vi "Sort Test Cases.vi"(10 "Test Cases":T1[](array[typedef]), 11 "Test Suites":string[](array[string])) -> (3 "Test Suites":T2[](array[typedef]))   [LabVIEW 2014, in "VI Tester Parsing.lvlib"]
uses:
  VI Tester Parsing.lvlib
  Test Suite.ctl
  Test Case.ctl
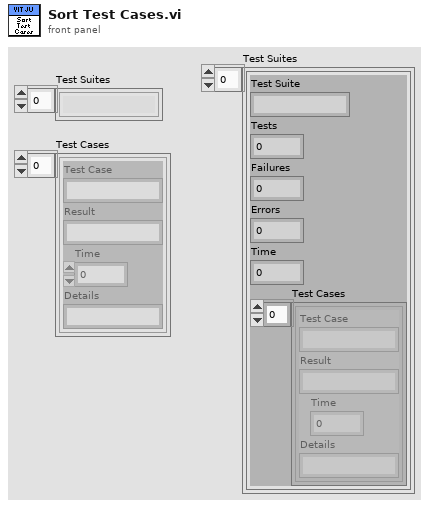
[diagram p1: front panel]
types:
  T1 = typedef "VI Tester Parsing.lvlib/Test Case.ctl" = cluster{"Test Case":string, "Result":string, "Time":dbl, "Details":string}
  T2 = typedef "VI Tester Parsing.lvlib/Test Suite.ctl" = cluster{"Test Suite":string, "Tests":i32, "Failures":i32, "Errors":i32, "Time":dbl, "Test Cases":T1[]}
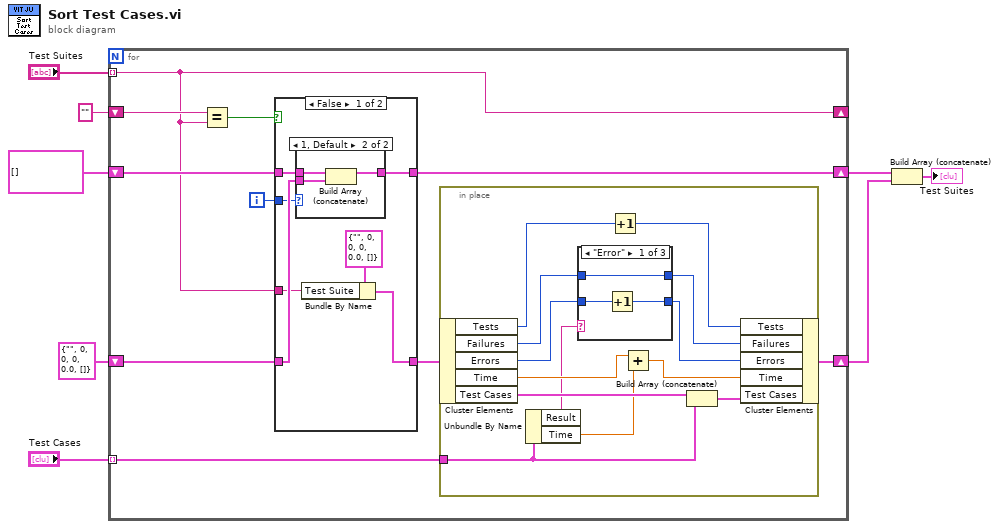
[diagram p0: block diagram]
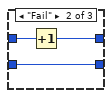
[diagram p2: hidden frame]
diagram:
  n1 = for {
    tunnel: "Test Cases" -> [w17] mode=indexing
    shift-right: [w9] -> _
    shift-left: "" -> [w10]
    shift-right: [w11] -> w6
    shift-left: T2 {"Test Suite"="", "Tests"=0, "Failures"=0, "Errors"=0, "Time"=0.0, "Test Cases"=[]} ("cluster") -> [w16]
    tunnel: "Test Suites" -> [w9] mode=indexing
    shift-right: [w14] -> w5
    shift-left: T2[] [] -> [w15]
    i -> [w12]
    n2 = Equal?(x=w10, y=w9) -> (x = y?=w18:bool)
    n3 = case shown="False" w18 {
      tunnel: w16 -> [w44 w52]
      tunnel: [w43 w52] -> w13
      tunnel: w15 -> [w46 w51]
      tunnel: [w45 w51] -> w14
      tunnel: w9 -> [w42 _]
      tunnel: w12 -> [w41 _]
      frame False {
        n4 = case shown="1, Default" w41 {
          tunnel: w46 -> [w47 w50]
          tunnel: [w47 w49] -> w45
          tunnel: w44 -> [_ w48]
          frame 0 {
          }
          frame 1, Default {
            n5 = Build Array (concatenate)(w50, w48) -> (w49:T2[])
          }
        }
        n6 = Bundle By Name(cluster=T2 {"Test Suite"="", "Tests"=0, "Failures"=0, "Errors"=0, "Time"=0.0, "Test Cases"=[]}, "Test Suite"=w42) -> (w43:T2)
      }
      frame True {
      }
    }
    n7 = in-place {
      in-place-border: w17 -> [w29]
      n8 = in-place-cluster #1(w13) -> ("Tests"=w22:i32, "Failures"=w24:i32, "Errors"=w20:i32, "Time"=w27:dbl, "Test Cases"=w31:T1[])
      n9 = Unbundle By Name(w29) -> ("Result"=w25:string, "Time"=w26:dbl)
      n10 = case shown="\"Error\"" w25 {
        tunnel: w24 -> [w34 w37 w39]
        tunnel: [w34 w36 w39] -> w23
        tunnel: w20 -> [w33 w35 w38]
        tunnel: [w32 w35 w38] -> w19
        frame "Error" {
          n11 = Increment(x=w33) -> (x+1=w32:i32)
        }
        frame "Fail" {
          n12 = Increment(x=w37) -> (x+1=w36:i32)
        }
        frame "Pass", Default {
        }
      }
      n13 = Increment(x=w22) -> (x+1=w21:i32)
      n14 = Add(x=w27, y=w26) -> (x+y=w28:dbl)
      n15 = Build Array (concatenate)(w31, w29) -> (w30:T1[])
      n16 = in-place-cluster #1("Tests"=w21, "Failures"=w23, "Errors"=w19, "Time"=w28, "Test Cases"=w30) -> (w11:T2)
    }
  }
  n17 = Build Array (concatenate)(w5, w6) -> (→"Test Suites":T2[])
